vi "FABR-Init Hardware.vi"(0 "Params":T3={"Stimulus"={"Destination"="", "Rep rate (/sec)"=25000.0, "Alternate Polarity"=FALSE, "Duration (ms)"=5.0, "Ramp (ms)"=0.0, "Fs (Hz)"=5.0, "Frame size (s)"=0.0}, "Sequence"={"Freq"={"Start (kHz)"=20.0, "Stop (kHz)"=80.0, "Step (oct)"=5.0, "Skip (oct)"=0.0}, "Level"={"Start (dB)"=20, "Stop (dB)"=80, "Step (dB)"=5}, "Order"=enum."Interleaved"}, "Response"={"Gain"=10000.0, "Averages"=512, "Window (ms)"=8.5, "Fs (Hz)"=25000.0, "Save raw"=FALSE}, "Reject"=0.5} {"Sequence"."Level"."Start (dB)" step=5; "Sequence"."Freq"."Start (kHz)" step=5.0; "Response"."Window (ms)" format="%.2f"}, 11 "error in (no error)":errorcluster) -> (8 "Runtime":T1, 10 "AO npts":i32, 15 "error out":errorcluster)   [LabVIEW 2020]
uses:
  Typedefs/FABR-Parameters.ctl
  Typedefs/FABR-Stimulus.ctl
  Typedefs/FABR-Sequence.ctl
  Typedefs/FABR-Order.ctl
  Typedefs/FABR-Response.ctl
  Typedefs/FABR-Runtime Data.ctl
  Typedefs/FABR-Stimulus Ticket.ctl
  e5209c82-ccee-4d4c-864f-4c40833b798d.vi
  0d666dbc-ef0b-4d81-a1c6-cd64144e6b2b.vi
  29bc1564-6995-4207-bd9a-3338b070ede7.vi
  9553b85a-16d4-40d0-9d08-d30bce0f45cc.vi
  <vilib>/Utility/config.llb/Open Config Data.vi
  <vilib>/Utility/config.llb/Get Key Names.vi
  <vilib>/Utility/config.llb/Read Key.vi
  <vilib>/Utility/config.llb/Read Key (String).vi
  epl-vi-lib/Utility VIs/Array Manipulation VIs/String Array to Comma Separated String.vi
  <vilib>/Utility/error.llb/Error Cluster From Error Code.vi
  <vilib>/Utility/config.llb/Close Config Data.vi
  epl-vi-lib/PXI DAQ VIs/AODO/AODO-Engine.vi
  epl-vi-lib/PXI DAQ VIs/AIDI/AIDI-Engine.vi
panel:
  out "Coerced rep rate":dbl
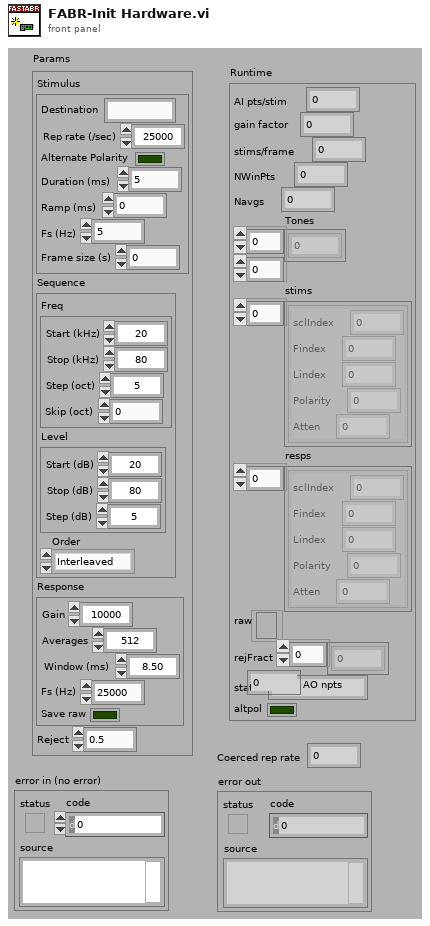
[diagram p1: front panel]
types:
  T1 = typedef "FABR-Runtime Data.ctl" = cluster{"AI pts/stim":i32, "gain factor":dbl, "stims/frame":i32, "NWinPts":i32, "Navgs":i32, "Tones":dbl[][], "stims":T2[], "resps":T2[], "raw":refnum<file>, "rejFract":dbl[], "status":string, "altpol":bool}
  T2 = typedef "FABR-Stimulus Ticket.ctl" = cluster{"sclIndex":i32, "Findex":i32, "Lindex":i32, "Polarity":i32, "Atten":dbl}
  T3 = typedef "FABR-Parameters.ctl" = cluster{"Stimulus":T4, "Sequence":T5, "Response":T7, "Reject":dbl}
  T4 = typedef "FABR-Stimulus.ctl" = cluster{"Destination":string, "Rep rate (/sec)":dbl, "Alternate Polarity":bool, "Duration (ms)":dbl, "Ramp (ms)":dbl, "Fs (Hz)":dbl, "Frame size (s)":dbl}
  T5 = typedef "FABR-Sequence.ctl" = cluster{"Freq":cluster{"Start (kHz)":dbl, "Stop (kHz)":dbl, "Step (oct)":dbl, "Skip (oct)":dbl}, "Level":cluster{"Start (dB)":i32, "Stop (dB)":i32, "Step (dB)":i32}, "Order":T6}
  T6 = typedef "FABR-Order.ctl" = enum16{"Interleaved"}
  T7 = typedef "FABR-Response.ctl" = cluster{"Gain":dbl, "Averages":i32, "Window (ms)":sgl, "Fs (Hz)":dbl, "Save raw":bool}
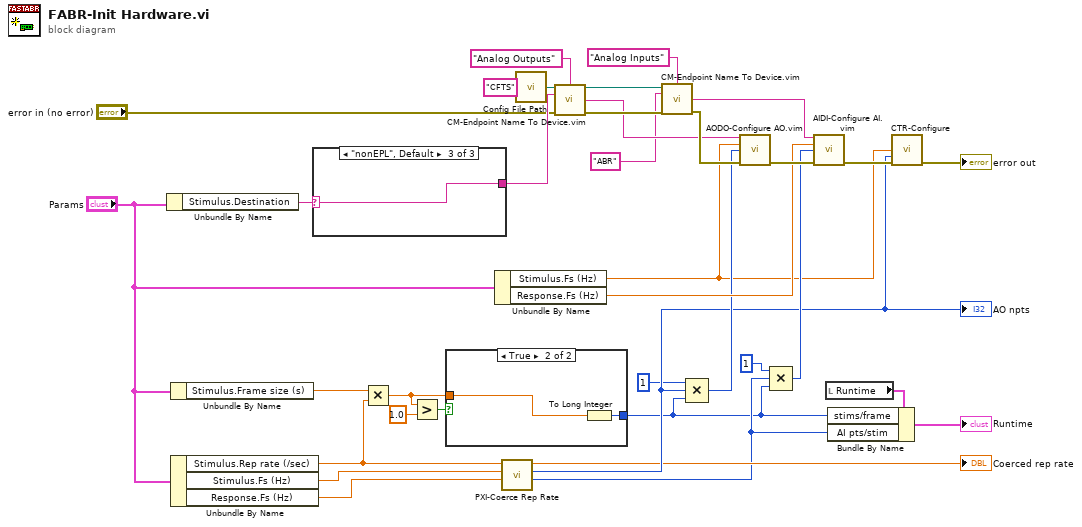
[diagram p0: block diagram]
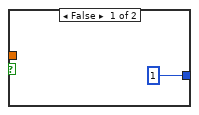
[diagram p2: hidden frame]
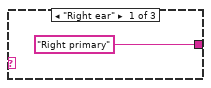
[diagram p3: hidden frame]
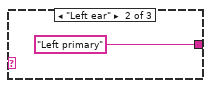
[diagram p4: hidden frame]
diagram:
  n1 = Unbundle By Name("Params") -> ("Stimulus.Destination"=w31:string)
  n2 = Unbundle By Name("Params") -> ("Stimulus.Frame size (s)"=w3:dbl)
  n3 = Unbundle By Name("Params") -> ("Stimulus.Rep rate (/sec)"=w32:dbl, "Stimulus.Fs (Hz)"=w18:dbl, "Response.Fs (Hz)"=w17:dbl)
  n4 = case shown="\"nonEPL\", Default" w31 {
    selector: w31 -> [_ _ w39]
    tunnel: ["Right primary" "Left primary" w39] -> w25
    frame "Right ear" {
    }
    frame "Left ear" {
    }
    frame "nonEPL", Default {
    }
  }
  n5 = Multiply(x=w3, y=w32) -> (x*y=w1:dbl)
  n6 = Greater?(x=w1, y=1.0) -> (0:w33:bool)
  n7 = case shown="True" w33 {
    tunnel: w1 -> [_ w41]
    tunnel: [1 w42] -> w4
    frame False {
    }
    frame True {
      # "next multiple of 10"
      n8 = To Long Integer(number=w41) -> (32bit integer=w42:i32)
    }
  }
  n9 = Unbundle By Name("Params") -> ("Stimulus.Fs (Hz)"=w9:dbl, "Response.Fs (Hz)"=w19:dbl)
  n10 = call "PXI-Coerce Rep Rate.vi"("AI sampling rate (Hz)"=w17, "AO sampling rate (Hz)"=w18, "Rep rate (Hz)"=w32) -> ("AI npts"=w5:i32, "AO npts"=w13:i32, "Coerced rep rate (Hz)"=→"Coerced rep rate":dbl)  [unwired: 5 in, 1 out]
  "AO npts" <- w13
  n11 = call "Config File Path.vi"("AppName"="CFTS") -> ("Default config file name"=w29:path)
  n12 = call "CM-Endpoint Name To Device.vim"("Path"=w29, "IO Type"="Analog Outputs", "Names in"=w25, "error in (no error)"="error in (no error)") -> ("Path thru"=w26:path, "Devices"=w22:string, "error out"=w24:errorcluster)  [unwired: 8 in, 1 out]
  n13 = call "CM-Endpoint Name To Device.vim"("Path"=w26, "IO Type"="Analog Inputs", "Names in"="ABR", "error in (no error)"=w24) -> ("Devices"=w20:string, "error out"=w23:errorcluster)  [unwired: 8 in, 2 out]
  n14 = Compound Arithmetic op=MULTIPLY(1 ("value"), w13, w4) -> (w16:i32)
  n15 = call "AODO-Configure AO.vim"("AO.Channels"=w22, "AO.Fs (Hz)"=w9, "AO.Npts"=w16, "error in (no error)"=w23) -> ("error out"=w21:errorcluster)  [unwired: 11 in]
  n16 = Compound Arithmetic op=MULTIPLY(1 ("value"), w5, w4) -> (w15:i32)
  n17 = call "AIDI-Configure AI.vim"("AI.Channels"=w20, "AI.Fs (Hz)"=w19, "AI.Npts"=w15, "error in (no error)"=w21) -> ("error out"=w14:errorcluster)  [unwired: 11 in]
  n18 = local read "Runtime"() -> (w36:T1)
  n19 = Bundle By Name(cluster=w36, "stims/frame"=w4, "AI pts/stim"=w5) -> (→"Runtime":T1)
  n20 = call "CTR-Configure.vi"("Sampling rate (Hz)"=w9, "Npts"=w13, "error in (no error)"=w14) -> ("error out"=→"error out":errorcluster)  [unwired: 12 in]
